vi "InitLog.vi"(6 "Compress old logs (F)":bool, 7 "disable buffering? (F)":bool, 8 "error in":errorcluster, 9 "Override file (F)":bool=TRUE, 10 "Default log level (info)":T2(ring)=enum."info", 11 "base path":path) -> (0 "error out":errorcluster, 3 "logger":T1)   [LabVIEW 2019]
doc: "Creates a log file (latest.log.tdms) in the base path specified. If Override file is false, then old files are moved to the format of <date>.tdms"
uses:
  Logger.ctl
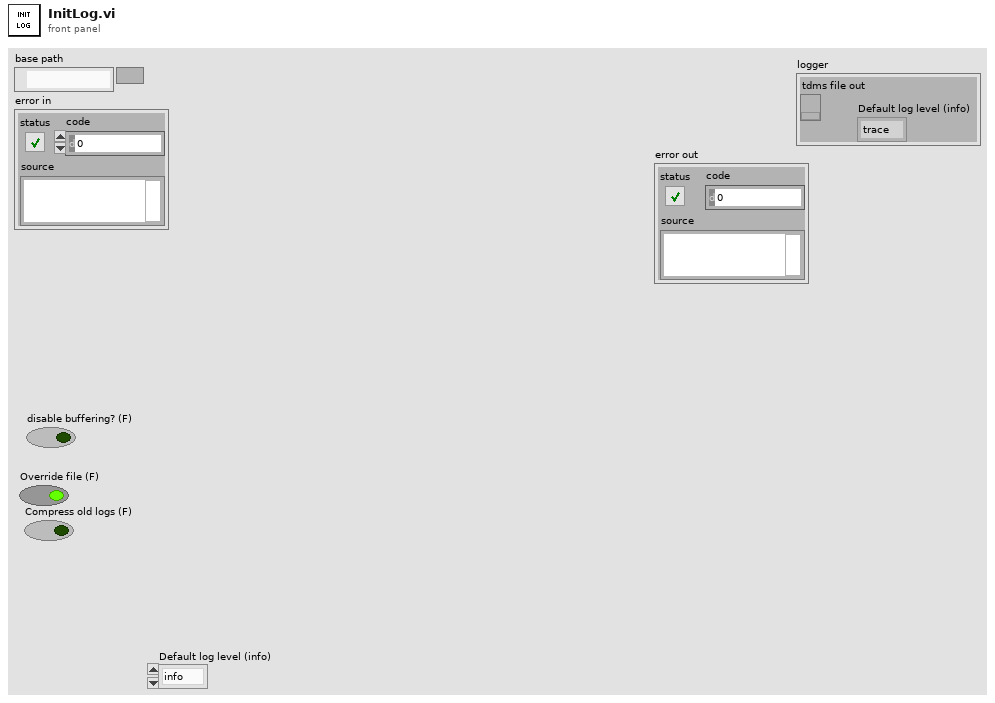
[diagram p1: front panel]
types:
  T1 = typedef "Logger.ctl" = cluster{"tdms file out":refnum<k34>, "Default log level (info)":enum16{"trace", "debug", "info", "warn", "error"}}
  T2 = enum16{"trace", "debug", "info", "warn", "error"}
  T3 = enum16{"open", "open or create", "create or replace", "create", "open (read-only)"}
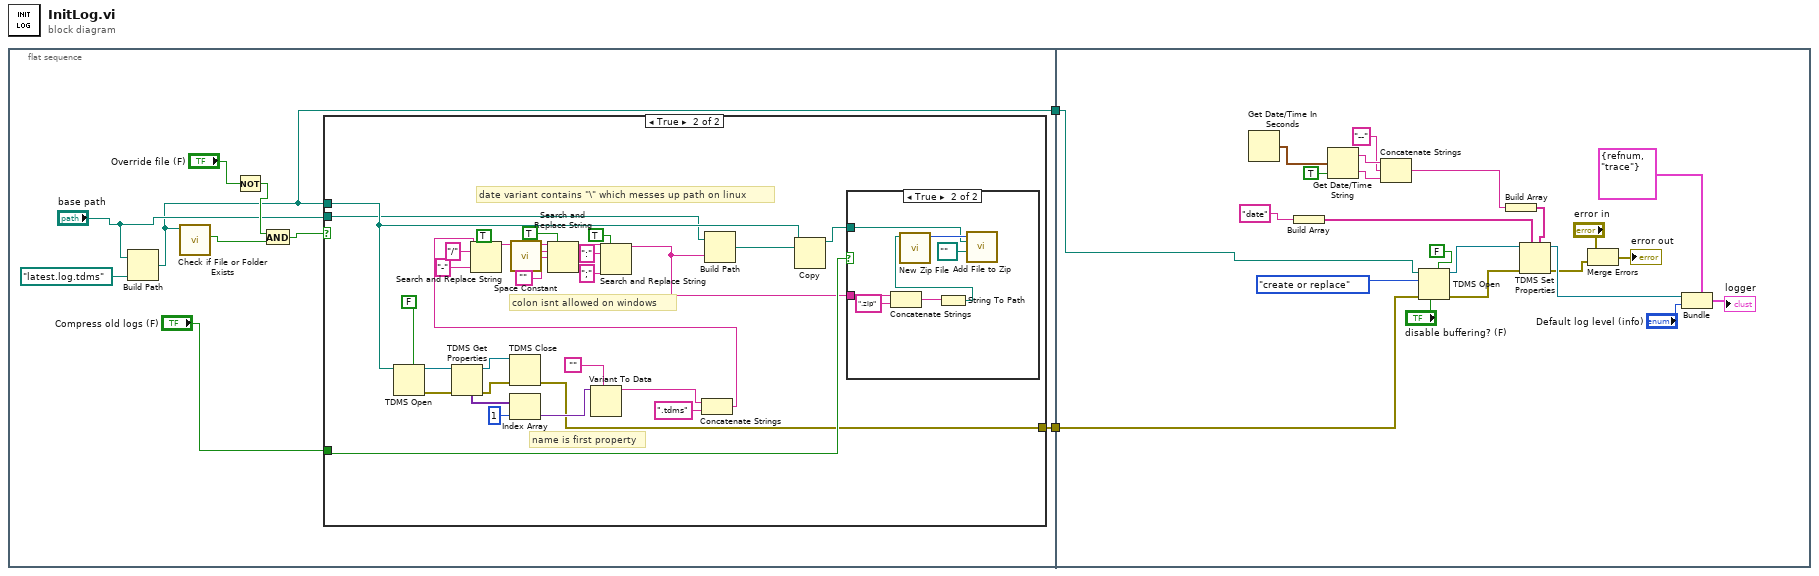
[diagram p0: block diagram]
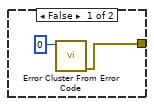
[diagram p2: hidden frame]
diagram:
  n1 = flat-sequence {
    tunnel: [w4] -> w2
    tunnel: [w3] -> w1
    tunnel: w2 -> [w63]
    tunnel: w1 -> [w54]
    frame #0 {
      n2 = Build Path(base path="base path", name or relative path=path "latest.log.tdms" ("path")) -> (appended path=w4:path)
      n3 = call <vilib>:"Check if File or Folder Exists.vi"("path"=w4) -> ("file or folder exists?"=w9:bool)  [unwired: 8 in, 2 out]
      n4 = Not(x="Override file (F)") -> (.not. x?=w10:bool)
      n5 = And(x=w10, y=w9) -> (x .and. y?=w11:bool)
      n6 = case shown="True" w11 {
        tunnel: "Compress old logs (F)" -> [_ w35]
        tunnel: w4 -> [_ w33]
        tunnel: "base path" -> [_ w31]
        tunnel: [w12 w14] -> w3
        frame False {
          n7 = call <vilib>:"Error Cluster From Error Code.vi"("error code (0)"=0) -> ("error out"=w12:errorcluster)  [unwired: 8 in]
        }
        frame True {
          # "colon isnt allowed on windows"
          # "date variant contains \"\\\" which messes up path on linux"
          # "name is first property"
          n8 = TDMS Open(5:FALSE ("create index file? (T)"), 11:w33) -> (0:w16:errorcluster, 3:w42:refnum<k34>)  [unwired: 5 in]
          n9 = TDMS Get Properties(8:w16, 11:w42) -> (0:w15:errorcluster, 3:w22:refnum<k34>, 4:w41:variant[])  [unwired: 4 in, 3 out]
          n10 = TDMS Close(8:w15, 11:w22) -> (0:w14:errorcluster)  [unwired: 1 out]
          n11 = Index Array(array=w41, index=1) -> (element=w39:variant)
          n12 = call <vilib>:"Space Constant.vi"() -> ("String"=w25:string)
          n13 = Variant To Data(type="", Variant=w39) -> (data=w36:string)  [unwired: 1 in, 1 out]
          n14 = Concatenate Strings(w36, ".tdms" ("string")) -> (w30:string)
          n15 = Search and Replace String(replace all?=TRUE ("replace all? (F)"), input string=w30, search string="/", replace string="-" ("replace string (\"\")")) -> (result string=w26:string)  [unwired: 4 in, 3 out]
          n16 = Search and Replace String(replace all?=TRUE ("replace all? (F)"), input string=w26, search string=w25, replace string="") -> (result string=w21:string)  [unwired: 4 in, 3 out]
          n17 = Search and Replace String(replace all?=TRUE ("replace all? (F)"), input string=w21, search string=":", replace string=";" ("replace string (\"\")")) -> (result string=w20:string)  [unwired: 4 in, 3 out]
          n18 = Build Path(base path=w31, name or relative path=w20) -> (appended path=w32:path)
          n19 = Copy(10:w32, 11:w33) -> (3:w34:path)  [unwired: 3 in, 2 out]
          n20 = case shown="True" w35 {
            tunnel: w34 -> [_ w46]
            tunnel: w20 -> [_ w45]
            frame False {
            }
            frame True {
              n21 = Concatenate Strings(w45, ".zip" ("string")) -> (w48:string)
              n22 = String To Path(string=w48) -> (path=w47:path)
              n23 = call <vilib>:"New Zip File.vi"("target"=w47) -> ("zip file out"=w50:i64)  [unwired: 4 in, 2 out]
              n24 = call <vilib>:"Add File to Zip.vi"("destination path in zip"=path "", "source file path"=w46, "zip file in"=w50) -> ()  [unwired: 7 in, 2 out]
            }
          }
        }
      }
    }
    frame #1 {
      n25 = Get Date/Time In Seconds() -> (seconds since 1Jan1904=w62:timestamp)
      n26 = Build Array("date") -> (w66:string[])
      n27 = Get Date/Time String(seconds (now)=w62, want seconds? (F)=TRUE) -> (date string=w61:string, time string=w59:string)  [unwired: 1 in]
      n28 = Concatenate Strings(w61, "--" ("string"), w59) -> (w58:string)
      n29 = TDMS Open(5:FALSE ("create index file? (T)"), 6:"disable buffering? (F)", 8:w54, 10:T3."create or replace" ("operation (0:open)"), 11:w63) -> (0:w55:errorcluster, 3:w72:refnum<k34>)  [unwired: 2 in]
      n30 = Build Array(w58) -> (w57:string[])
      n31 = TDMS Set Properties(5:w57, 7:w66, 8:w55, 11:w72) -> (0:w53:errorcluster, 3:w73:refnum<k34>)  [unwired: 2 in, 2 out]
      n32 = Merge Errors("error in", w53) -> (→"error out":errorcluster)
      n33 = Bundle(cluster=T1 {"tdms file out"=refnum, "Default log level (info)"=enum."trace"} ("logger"), "tdms file out"=w73, "Default log level (info)"="Default log level (info)") -> (→"logger":T1)
    }
  }
